vi "Get LeafNodeTempValues.vi"(8 "error in (no error)":errorcluster caption="错误输入（无错误）", 11 "PanelRootNode 输入":refnum<class "PanelRootNode.lvclass"> caption="DNL_LabVIEW Object in") -> (0 "error out":errorcluster caption="错误输出", 2 "TempValue":variant[](array[variant]), 3 "PanelRootNode 输出":refnum<class "PanelRootNode.lvclass"> caption="DNL_LabVIEW Object out")   [LabVIEW 2013, in "PanelRootNode.lvclass"]
uses:
  PanelRootNode.lvclass
  PanelDataNode/PanelDataNode.lvclass
  PanelDataNode/PanelDataNode.lvclass/PanelDataNode.ctl
panel:
  in  "PanelNumber(-1)":i32=-1
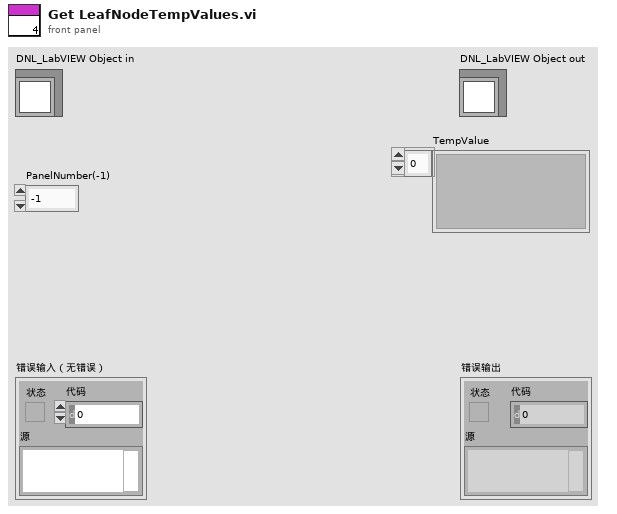
[diagram p1: front panel]
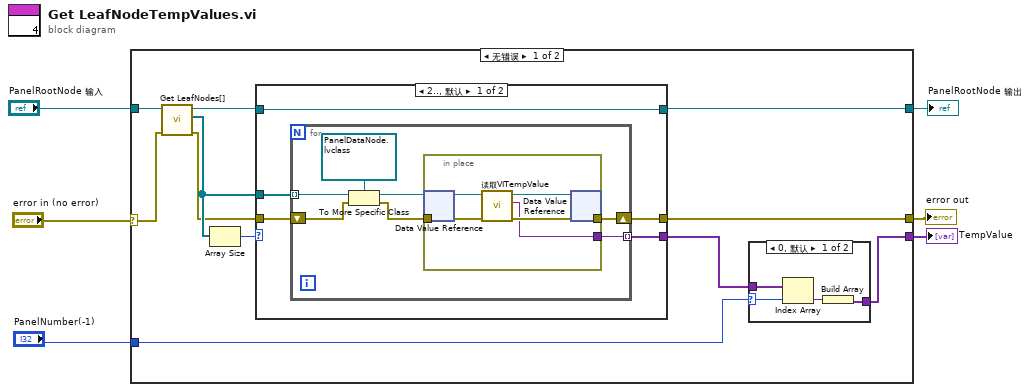
[diagram p0: block diagram]
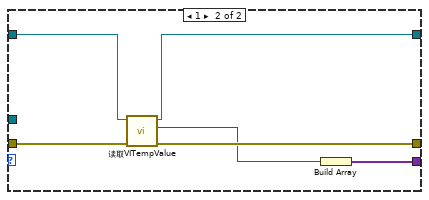
[diagram p3: hidden frame]
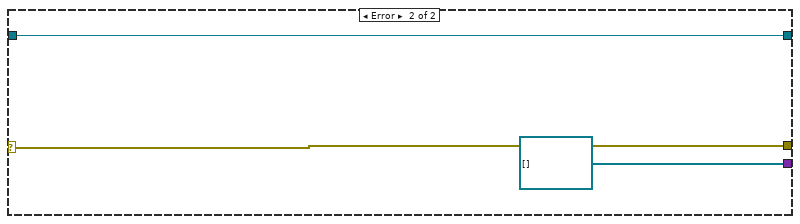
[diagram p4: hidden frame]
diagram:
  n1 = case shown="无错误" "error in (no error)" {
    selector: "error in (no error)" -> [w12 w48]
    tunnel: [w10 w48] -> w5
    tunnel: [w15 w47] -> w4
    tunnel: "PanelRootNode 输入" -> [w17 w47]
    tunnel: [w8 refnum<vi>[] []] -> w1
    tunnel: "PanelNumber(-1)" -> [w7 _]
    frame No Error {
      n2 = call "Get LeafNodes[].vi"("error in (no error)"=w12, "PanelRootNode 输入"=w17) -> ("error out"=w11:errorcluster, "LeafNodes[]"=w14:refnum<data-value>[], "PanelRootNode 输出"=w16:refnum<class "PanelRootNode.lvclass">)  [unwired: 7 in]
      n3 = Array Size(array=w14) -> (size(s)=w13:i32)
      n4 = case shown="2.., 默认" w13 {
        tunnel: w16 -> [w27 w44]
        tunnel: [w27 w43] -> w15
        tunnel: w14 -> [w26 _]
        tunnel: [w25 w45] -> w9
        tunnel: w11 -> [w24 w42]
        tunnel: [w23 w41] -> w10
        frame 2.., Default {
          n5 = for {
            tunnel: w26 -> [w33] mode=indexing
            tunnel: [w34] -> w25 mode=indexing
            shift-right: [w28] -> w23
            shift-left: w24 -> [w29]
            n6 = To More Specific Class(target class=refnum<data-value> refnum ("数据值引用"), reference=w33, error in=w29) -> (specific class reference=w32:refnum<data-value>, error out=w30:errorcluster)
            n7 = in-place {
              in-place-border: [w35] -> w34
              in-place-border: w30 -> [w37]
              in-place-border: [w36] -> w28
              n8 = in-place-dvr #1(w32) -> (w39:refnum<class "PanelDataNode.lvclass">)  [unwired: 1 out]
              n9 = call "读取VITempValue.vi"("error in (no error)"=w37, "PanelDataNode输入"=w39) -> ("error out"=w36:errorcluster, "VITempValue"=w35:variant, "PanelDataNode输出"=w38:refnum<class "PanelDataNode.lvclass">)  [unwired: 7 in]
              n10 = in-place-dvr #1(w38) -> ()  [unwired: 2 out]
            }
          }
        }
        frame 1 {
          n11 = call "读取VITempValue.vi"("error in (no error)"=w42, "PanelDataNode输入"=w44) -> ("error out"=w41:errorcluster, "VITempValue"=w40:variant, "PanelDataNode输出"=w43:refnum<class "PanelRootNode.lvclass">)  [unwired: 7 in]
          n12 = Build Array(w40) -> (w45:variant[])
        }
      }
      n13 = case shown="0, 默认" w7 {
        selector: w7 -> [w20 _]
        tunnel: w9 -> [w21 w22]
        tunnel: [w18 w22] -> w8
        frame 0, Default {
          n14 = Index Array(array=w21, index=w20) -> (element=w19:variant)
          n15 = Build Array(w19) -> (w18:variant[])
        }
        frame -1 {
        }
      }
    }
    frame Error {
    }
  }
  "error out" <- w5
  "PanelRootNode 输出" <- w4
  "TempValue" <- w1
